vi "VG_SOC.vi"() -> ()   [LabVIEW 2020]
panel:
  in  "SOC":string
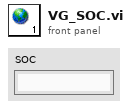
[diagram p1: front panel]
diagram:
